vi "save ROI.vi"() -> ()   [LabVIEW 2012]
panel:
  out "Save Coordinates":T1(array[cluster])
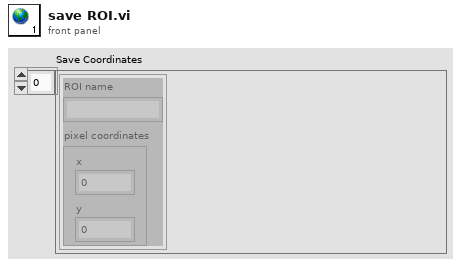
[diagram p1: front panel]
types:
  T1 = cluster{"ROI name":string, "pixel coordinates":cluster{"x":i32, "y":i32}}[]
diagram:
